vi "query.vi"(6 "ms timeout (0:default)":i32, 8 "error in (no error)":errorcluster, 9 "query":string, 10 "token in (random)":u64 format="%016x", 11 "rethinkdb in":T1) -> (0 "error out":errorcluster, 1 "response":string, 2 "token out":u64 format="%016x", 3 "rethinkdb out":T1)   [LabVIEW 2017, in "rethinkdb.lvlib"]
uses:
  rethinkdb.lvlib
  refnum.ctl
  private.ctl
  debug_fg.vi
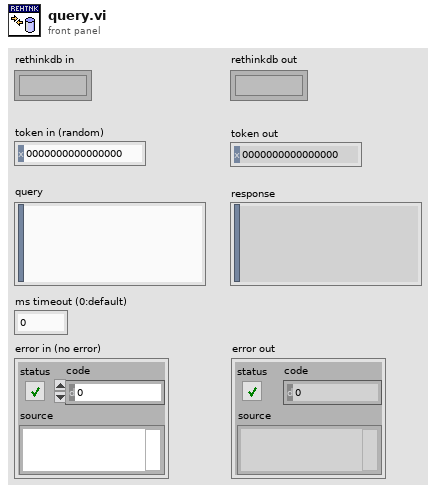
[diagram p1: front panel]
types:
  T1 = typedef "rethinkdb.lvlib/refnum.ctl" = refnum<k1>
  T2 = typedef "rethinkdb.lvlib/private.ctl" = cluster{"host":string, "port":u16, "user":string, "password":string, "ms_timeout":i32, "conn":refnum<k5>, "authentication":string}
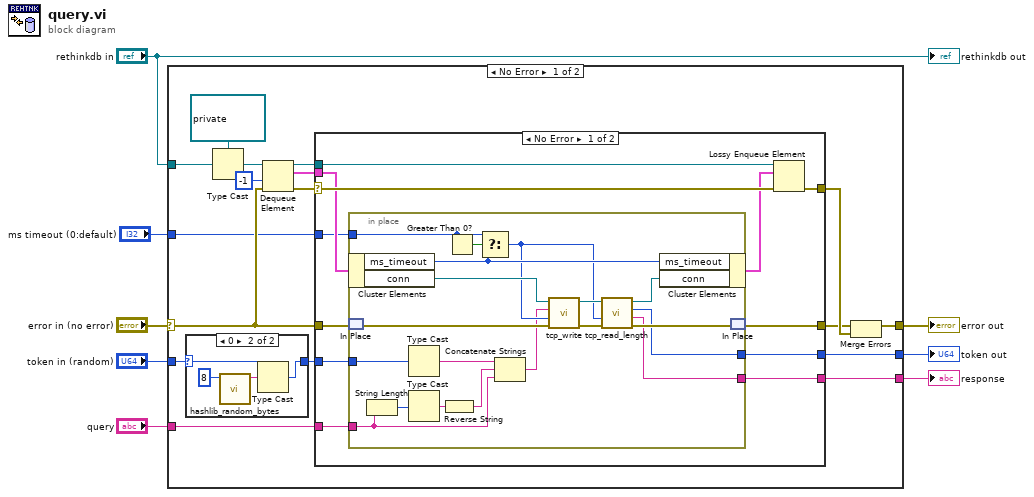
[diagram p0: block diagram]
diagram:
  n1 = case shown="No Error" "error in (no error)" {
    selector: "error in (no error)" -> [w17 w64]
    tunnel: "rethinkdb in" -> [w24 _]
    tunnel: [w16 w64] -> w6
    tunnel: "token in (random)" -> [w11 _]
    tunnel: "query" -> [w14 _]
    tunnel: [w13 _] -> w3
    tunnel: [w12 _] -> w2
    tunnel: "ms timeout (0:default)" -> [w9 _]
    frame No Error {
      n2 = case shown="0" w11 {
        selector: w11 -> [w26 w28]
        tunnel: [w26 w27] -> w10
        frame Default {
        }
        frame 0 {
          n3 = call "hashlib_random_bytes.vi"("length (18bytes)"=8 ("length")) -> ("random bytes"=w29:string)  [unwired: 10 in]
          n4 = Type Cast(type=w28, x=w29) -> (*(type *) &x=w27:u64)
        }
      }
      n5 = Type Cast(type=refnum<queue> refnum ("queue out"), x=w24) -> (*(type *) &x=w23:refnum<queue>)
      n6 = Dequeue Element(queue=w23, timeout in ms (-1)=-1, error in (no error)=w17) -> (queue out=w21:refnum<queue>, element=w20:T2, error out=w19:errorcluster)  [unwired: 1 out]
      n7 = case shown="No Error" w19 {
        selector: w19 -> [w41 w63]
        tunnel: w21 -> [w42 _]
        tunnel: w20 -> [w37 _]
        tunnel: [w40 w63] -> w18
        tunnel: w17 -> [w39 w62]
        tunnel: [w38 w62] -> w15
        tunnel: w10 -> [w35 _]
        tunnel: w14 -> [w34 _]
        tunnel: [w33 _] -> w13
        tunnel: [w32 _] -> w12
        tunnel: w9 -> [w31 _]
        frame No Error {
          n8 = in-place {
            in-place-border: w35 -> [w59]
            in-place-border: w34 -> [w58]
            in-place-border: [w53] -> w33
            in-place-border: [w52] -> w32
            in-place-border: w31 -> [w50]
            n9 = in-place-cluster #1(w37) -> ("ms_timeout"=w49:i32, "conn"=w48:refnum<k5>)
            n10 = in-place-match #2(w39) -> (w45:errorcluster)
            n11 = String Length(string=w58) -> (length=w54:i32)
            n12 = Type Cast(x=w59) -> (*(type *) &x=w56:string)  [unwired: 1 in]
            n13 = Type Cast(x=w54) -> (*(type *) &x=w55:string)  [unwired: 1 in]
            n14 = Reverse String(1:w55) -> (0:w57:string)
            n15 = Greater Than 0?(x=w50) -> (x > 0?=w51:bool)
            n16 = Select(t=w50, s=w51, f=w49) -> (s? t:f=w44:i32)
            n17 = Concatenate Strings(w56, w57, w58) -> (w43:string)
            n18 = call "tcp_write.vi"("error in (no error)"=w45, "ms_timeout"=w44, "data in"=w43, "conn in"=w48) -> ("error out"=w46:errorcluster, "conn out"=w47:refnum<k5>)  [unwired: 6 in]
            n19 = call "tcp_read_length.vi"("error in (no error)"=w46, "timeout ms (10000)"=w44, "conn in"=w47) -> ("error out"=w61:errorcluster, "response"=w52:string, "token"=w53:u64, "conn out"=w60:refnum<k5>)  [unwired: 5 in]
            n20 = in-place-cluster #1("ms_timeout"=w49, "conn"=w60) -> (w36:T2)
            n21 = in-place-match #2(w61) -> (w38:errorcluster)
          }
          n22 = Lossy Enqueue Element(queue=w42, element=w36, error in (no error)=w41) -> (error out=w40:errorcluster)  [unwired: 3 out]
        }
        frame Error {
        }
      }
      n23 = Merge Errors(w15, w18) -> (w16:errorcluster)
    }
    frame Error {
    }
  }
  "error out" <- w6
  "response" <- w2
  "token out" <- w3
  "rethinkdb out" <- "rethinkdb in"
